vi "PT3_IntArrayToImgHeader.vi"(11 "Array":i32[](array[numeric])) -> (2 "PI Header":bool, 3 "Image Header":T1)   [LabVIEW 2010]
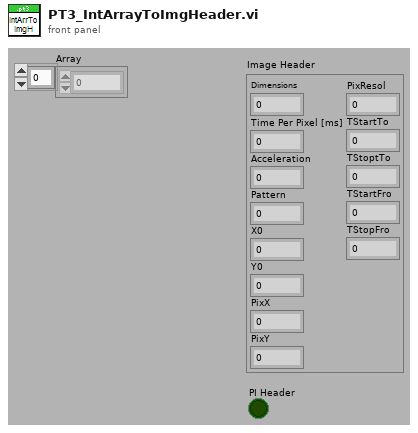
[diagram p1: front panel]
types:
  T1 = cluster{"Dimensions":i32, "Time Per Pixel [ms]":dbl, "Acceleration":i32, "Pattern":i32, "X0":sgl, "Y0":sgl, "PixX":i32, "PixY":i32, "PixResol":sgl, "TStartTo":sgl, "TStoptTo":sgl, "TStartFro":sgl, "TStopFro":sgl}
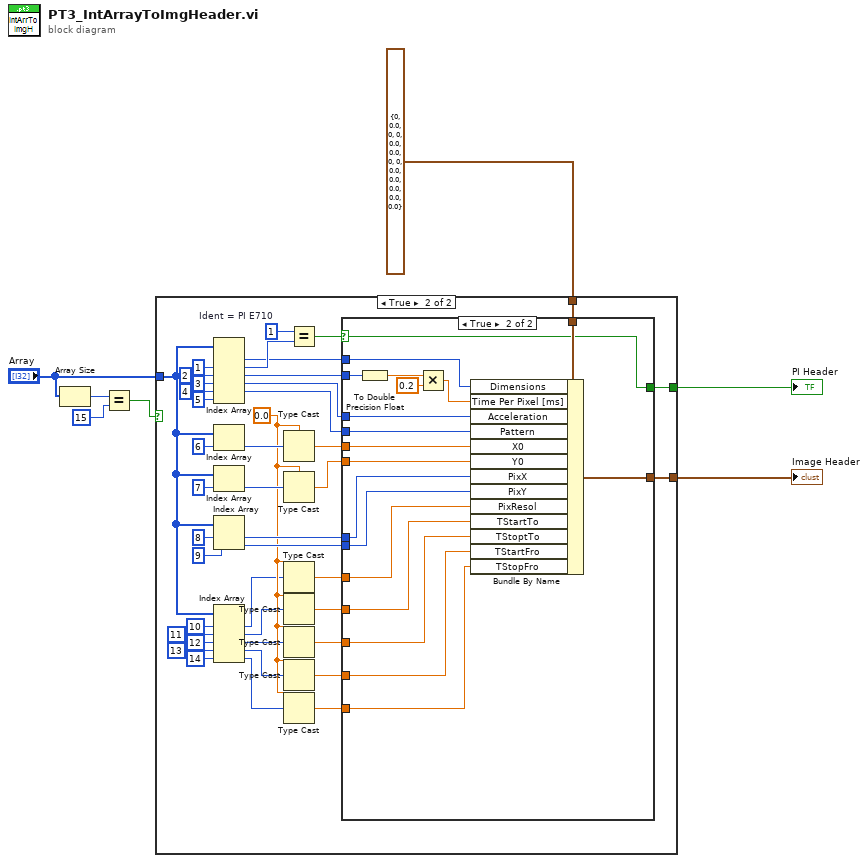
[diagram p0: block diagram]
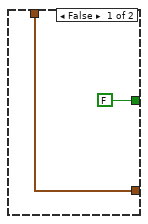
[diagram p2: hidden frame]
diagram:
  n1 = Array Size(array="Array") -> (size(s)=w6:i32)
  n2 = Equal?(x=w6, y=15) -> (x = y?=w4:bool)
  n3 = case shown="True" w4 {
    tunnel: "Array" -> [_ w40]
    tunnel: T1 {"Dimensions"=0, "Time Per Pixel [ms]"=0.0, "Acceleration"=0, "Pattern"=0, "X0"=0.0, "Y0"=0.0, "PixX"=0, "PixY"=0, "PixResol"=0.0, "TStartTo"=0.0, "TStoptTo"=0.0, "TStartFro"=0.0, "TStopFro"=0.0} ("Image Header") -> [w9 w31]
    tunnel: [w9 w30] -> w2
    tunnel: [FALSE w10] -> w1
    frame False {
    }
    frame True {
      w32 = 1  # Ident = PI E710
      w21 = sgl 0.0
      n4 = Index Array(array=w40, index #2=1 ("index"), index #3=2 ("index"), index #4=3 ("index"), index #5=4 ("index"), index #6=5 ("index")) -> (element #1=w29:i32, element #2=w34:i32, element #3=w28:i32, element #4=w27:i32, element #5=w26:i32)  [unwired: 1 in, 1 out]
      n5 = Index Array(array=w40, index=6) -> (element=w51:i32)
      n6 = Index Array(array=w40, index=7) -> (element=w48:i32)
      n7 = Index Array(array=w40, index #1=8 ("index"), index #2=9 ("index")) -> (element #1=w23:i32, element #2=w22:i32)
      n8 = Index Array(array=w40, index #1=10 ("index"), index #2=11 ("index"), index #3=12 ("index"), index #4=13 ("index"), index #5=14 ("index")) -> (element #1=w20:i32, element #2=w19:i32, element #3=w18:i32, element #4=w16:i32, element #5=w17:i32)
      n9 = Type Cast(type=w21, x=w51) -> (*(type *) &x=w25:sgl)
      n10 = Type Cast(type=w21, x=w48) -> (*(type *) &x=w24:sgl)
      n11 = Type Cast(type=w21, x=w20) -> (*(type *) &x=w15:sgl)
      n12 = Type Cast(type=w21, x=w19) -> (*(type *) &x=w12:sgl)
      n13 = Type Cast(type=w21, x=w18) -> (*(type *) &x=w13:sgl)
      n14 = Type Cast(type=w21, x=w16) -> (*(type *) &x=w11:sgl)
      n15 = Type Cast(type=w21, x=w17) -> (*(type *) &x=w14:sgl)
      n16 = Equal?(x=w32, y=w34) -> (x = y?=w33:bool)
      n17 = case shown="True" w33 {
        selector: w33 -> [w52 w54]
        tunnel: w31 -> [w53 w72]
        tunnel: [w53 w71] -> w30
        tunnel: w29 -> [_ w70]
        tunnel: w28 -> [_ w69]
        tunnel: w27 -> [_ w65]
        tunnel: w26 -> [_ w64]
        tunnel: w25 -> [_ w63]
        tunnel: w24 -> [_ w62]
        tunnel: w23 -> [_ w61]
        tunnel: w22 -> [_ w60]
        tunnel: w15 -> [_ w59]
        tunnel: w14 -> [_ w58]
        tunnel: w13 -> [_ w57]
        tunnel: w12 -> [_ w56]
        tunnel: w11 -> [_ w55]
        tunnel: [w52 w54] -> w10
        frame False {
        }
        frame True {
          n18 = To Double Precision Float(number=w69) -> (double precision float=w68:dbl)
          n19 = Multiply(x=w68, y=0.2) -> (x*y=w66:dbl)
          n20 = Bundle By Name(cluster=w72, "Dimensions"=w70, "Time Per Pixel [ms]"=w66, "Acceleration"=w65, "Pattern"=w64, "X0"=w63, "Y0"=w62, "PixX"=w61, "PixY"=w60, "PixResol"=w59, "TStartTo"=w56, "TStoptTo"=w57, "TStartFro"=w55, "TStopFro"=w58) -> (w71:T1)
        }
      }
    }
  }
  "Image Header" <- w2
  "PI Header" <- w1
